vi "dfd_Convert String to Numeric Array.vi"(8 "error in":errorcluster, 11 "string":string) -> (0 "error out":errorcluster, 3 "numeric array":dbl[](array[numeric]))   [LabVIEW 2017, in "NI_DigFilter_Process.lvlib"]
uses:
  <vilib>/addons/Digital Filter Design/NI_DigFilter_Process.lvlib
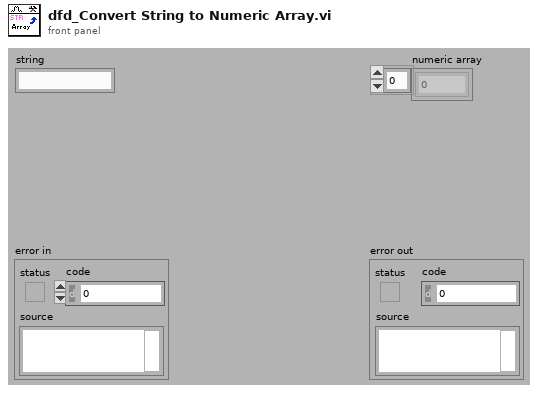
[diagram p1: front panel]
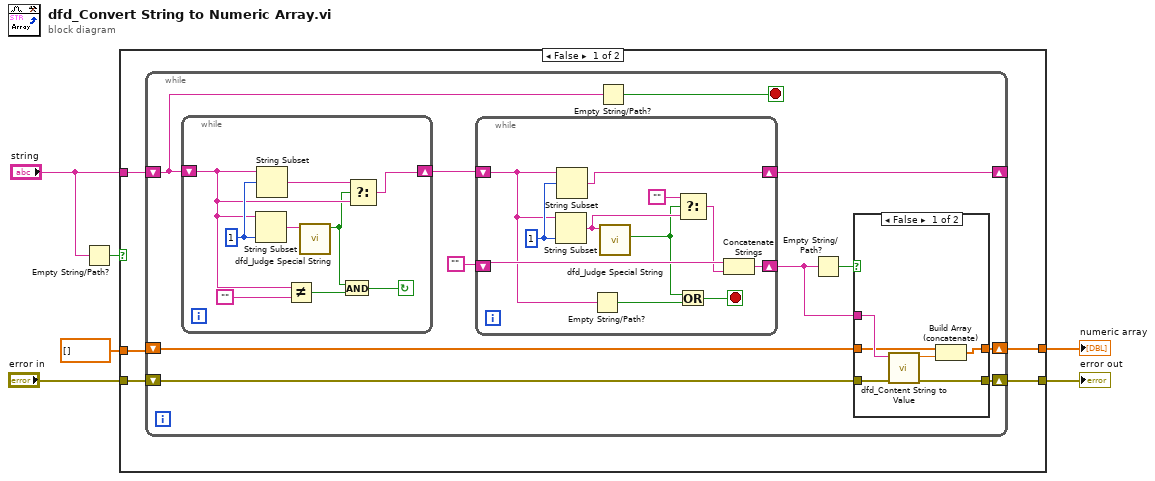
[diagram p0: block diagram]
diagram:
  n1 = Empty String/Path?(string/path="string") -> (empty?=w2:bool)
  n2 = case shown="False" w2 {
    tunnel: "string" -> [w11 _]
    tunnel: [w10 w52] -> w6
    tunnel: "error in" -> [w9 w51]
    tunnel: [w8 w51] -> w4
    tunnel: dbl[] [] -> [w7 w52]
    frame False {
      n3 = while {
        shift-right: [w22] -> _
        shift-left: w11 -> [w19]
        shift-right: [w15] -> w8
        shift-left: w9 -> [w14]
        shift-right: [w13] -> w10
        shift-left: w7 -> [w12]
        stop <- w18 stop-if-true
        n4 = while {
          shift-right: [w48] -> w21
          shift-left: w19 -> [w46]
          stop <- w43 continue-if-true
          w50 = 1 ("length (rest)")
          n5 = String Subset(string=w46, length (rest)=w50) -> (substring=w47:string)  [unwired: 1 out]
          n6 = String Subset(string=w46, offset (0)=w50) -> (substring=w49:string)  [unwired: 1 out]
          n7 = Not Equal?(x=w46, y="") -> (x != y?=w45:bool)
          n8 = call <vilib>:"dfd_Judge Special String.vi"("string"=w47) -> ("space ?"=w44:bool)  [unwired: 10 out]
          n9 = And(x=w44, y=w45) -> (x .and. y?=w43:bool)
          n10 = Select(t=w49, s=w44, f=w46) -> (s? t:f=w48:string)
        }
        n11 = while {
          shift-right: [w39] -> w22
          shift-left: w21 -> [w34]
          shift-right: [w35] -> w16
          shift-left: "" -> [w40]
          stop <- w31 stop-if-true
          w41 = 1 ("length (rest)")
          n12 = String Subset(string=w34, length (rest)=w41) -> (substring=w38:string)  [unwired: 1 out]
          n13 = String Subset(string=w34, offset (0)=w41) -> (substring=w39:string)  [unwired: 1 out]
          n14 = Empty String/Path?(string/path=w34) -> (empty?=w33:bool)
          n15 = call <vilib>:"dfd_Judge Special String.vi"("string"=w38) -> ("separator"=w32:bool)  [unwired: 10 out]
          n16 = Select(t="", s=w32, f=w38) -> (s? t:f=w37:string)
          n17 = Or(x=w32, y=w33) -> (x .or. y?=w31:bool)
          n18 = Concatenate Strings(w40, w37) -> (w35:string)
        }
        n19 = Empty String/Path?(string/path=w19) -> (empty?=w18:bool)
        n20 = Empty String/Path?(string/path=w16) -> (empty?=w17:bool)
        n21 = case shown="False" w17 {
          tunnel: w16 -> [w27 _]
          tunnel: [w26 w29] -> w15
          tunnel: w14 -> [w25 w29]
          tunnel: [w24 w30] -> w13
          tunnel: w12 -> [w23 w30]
          frame False {
            n22 = call <vilib>:"dfd_Content String to Value.vi"("error in (no error)"=w25, "string"=w27) -> ("error out"=w26:errorcluster, "value"=w28:dbl)  [unwired: 8 out]
            n23 = Build Array (concatenate)(w23, w28) -> (w24:dbl[])
          }
          frame True {
          }
        }
      }
    }
    frame True {
    }
  }
  "numeric array" <- w6
  "error out" <- w4
